vi "Write RGB.vi"(8 "error in (no error)":errorcluster, 10 "Color Box":u32(colorbox), 11 "Grove I2C RGB SGM31323 in":refnum<class "Grove I2C RGB SGM31323.lvclass">) -> (0 "error out":errorcluster, 3 "Grove I2C RGB SGM31323 out":refnum<class "Grove I2C RGB SGM31323.lvclass">)   [LabVIEW 2020, in "CTI-Peripheral.lvlib" / "Grove I2C RGB SGM31323.lvclass"]
uses:
  Grove I2C RGB SGM31323.lvclass
  Grove I2C RGB SGM31323.lvclass/Grove I2C RGB SGM31323.ctl
  CTI/I2C Connection/I2C Connection.lvclass/I2C Connection.ctl
  CTI/Session/I2C Write Data.vi
  CTI/I2C Connection/I2C Connection.lvclass
panel:
  out "blue":u8=250
  out "Green":u8=250
  out "Red":u8=250
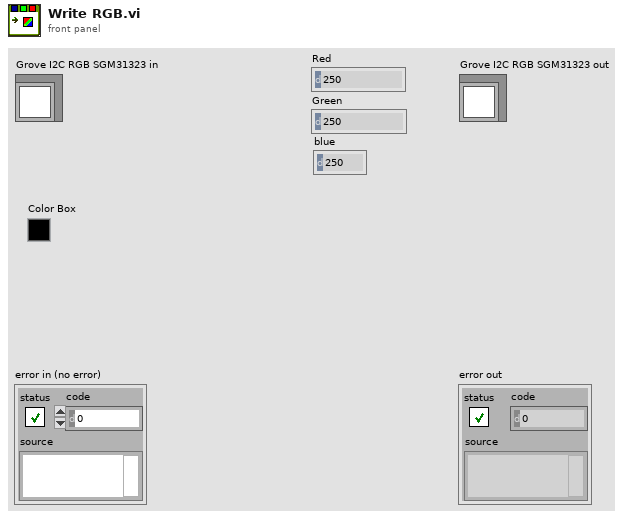
[diagram p1: front panel]
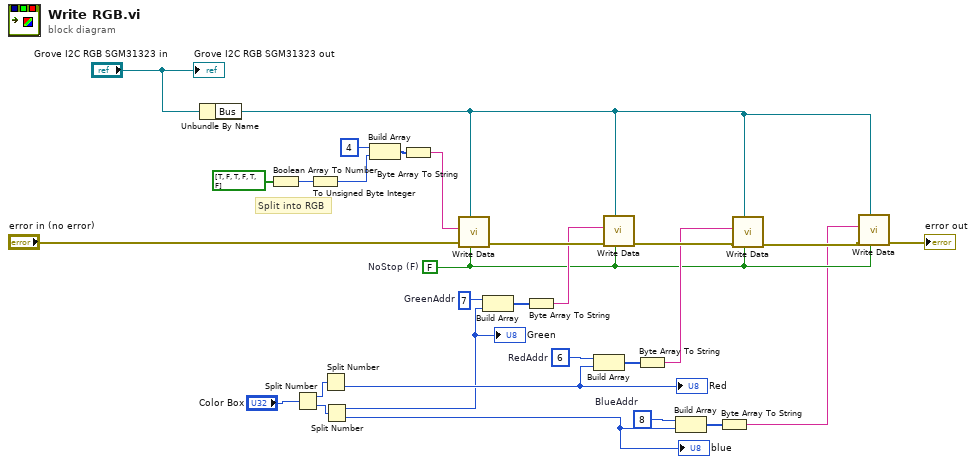
[diagram p0: block diagram]
diagram:
  w3 = FALSE  # NoStop (F)
  w24 = u8 8  # BlueAddr
  w26 = u8 7  # GreenAddr
  w28 = u8 6  # RedAddr
  # "Split into RGB"
  n1 = Unbundle By Name("Grove I2C RGB SGM31323 in") -> ("Bus"=w4:refnum<class "I2C Connection.lvclass">)
  n2 = Boolean Array To Number(Boolean array=bool[] [TRUE, FALSE, TRUE, FALSE, TRUE, FALSE] ("Array")) -> (number=w15:u32)
  n3 = Split Number(x="Color Box") -> (hi(x)=w22:u16, lo(x)=w23:u16)
  n4 = To Unsigned Byte Integer(number=w15) -> (unsigned 8bit integer=w16:u8)
  n5 = Split Number(x=w22) -> (lo(x)=w21:u8)  [unwired: 1 out]
  "Red" <- w21
  n6 = Split Number(x=w23) -> (hi(x)=w20:u8, lo(x)=w19:u8)
  "Green" <- w20
  "blue" <- w19
  n7 = Build Array(u8 4 ("Value"), w16) -> (w12:u8[])
  n8 = Byte Array To String(unsigned byte array=w12) -> (string=w11:string)
  n9 = call "Write Data.vi"("NoStop (F)"=w3, "I2C Connection"=w4, "error in (no error)"="error in (no error)", "Data"=w11) -> ("error out"=w10:errorcluster)  [unwired: 7 in]
  n10 = Build Array(w26, w20) -> (w29:u8[])
  n11 = Byte Array To String(unsigned byte array=w29) -> (string=w8:string)
  n12 = Build Array(w28, w21) -> (w27:u8[])
  n13 = call "Write Data.vi"("NoStop (F)"=w3, "I2C Connection"=w4, "error in (no error)"=w10, "Data"=w8) -> ("error out"=w7:errorcluster)  [unwired: 7 in]
  n14 = Byte Array To String(unsigned byte array=w27) -> (string=w6:string)
  n15 = Build Array(w24, w19) -> (w25:u8[])
  n16 = Byte Array To String(unsigned byte array=w25) -> (string=w2:string)
  n17 = call "Write Data.vi"("NoStop (F)"=w3, "I2C Connection"=w4, "error in (no error)"=w7, "Data"=w6) -> ("error out"=w5:errorcluster)  [unwired: 7 in]
  n18 = call "Write Data.vi"("NoStop (F)"=w3, "I2C Connection"=w4, "error in (no error)"=w5, "Data"=w2) -> ("error out"=→"error out":errorcluster)  [unwired: 7 in]
  "Grove I2C RGB SGM31323 out" <- "Grove I2C RGB SGM31323 in"
